vi "swabian_apply_channel_settings.vi"(8 "error in (no error)":errorcluster, 9 "Trigger edge":bool[](array[boolean])=[FALSE, FALSE, FALSE, FALSE, FALSE, FALSE, FALSE, FALSE], 10 "swabian_channel_settings":T5=[{"Threshold (V)"=0.5, "Input Delay (ps)"=0, "Dead Time (ps)"=6000}, {"Threshold (V)"=0.5, "Input Delay (ps)"=0, "Dead Time (ps)"=6000}, {"Threshold (V)"=0.5, "Input Delay (ps)"=0, "Dead Time (ps)"=6000}, {"Threshold (V)"=0.5, "Input Delay (ps)"=0, "Dead Time (ps)"=6000}, {"Threshold (V)"=0.5, "Input Delay (ps)"=0, "Dead Time (ps)"=6000}, {"Threshold (V)"=0.5, "Input Delay (ps)"=0, "Dead Time (ps)"=6000}, {"Threshold (V)"=0.5, "Input Delay (ps)"=0, "Dead Time (ps)"=6000}, {"Threshold (V)"=0.5, "Input Delay (ps)"=0, "Dead Time (ps)"=6000}] {"Dead Time (ps)" min=0 step=6000; "Input Delay (ps)" min=0 step=1; "Threshold (V)" min=0.0 max=2.5 step=0.1}, 11 "swabian_local_data":T1={"events"={"update_status"=refnum, "update_chart"=refnum, "update_xy"=refnum, "send_channel_data"=refnum}, "stop_q"=refnum, "tagger_reference"=refnum, "connect_button"=refnum, "counter_reference"=refnum, "tagger_stream_reference"=refnum, "log_reference"=refnum, "current_log_offset"=0, "tt20_buffer_q"=refnum, "stream_to_file_button"=refnum, "num_records"=0, "connected?"=FALSE, "plots"=refnum, "histogram_bin_edges"=[], "histogrammer"=refnum, "plot_lifetimes"=refnum, "xy_graph"=refnum, "Reference\nChannel"=enum."ch0", "trigger_channels"=[], "filter_channels"=[], "active_channels"=[], "acq_mode"=0, "Reference\nChannel"=enum."ch0", "acq_time"=0, "leftovers"={"leftover_stamps"=[], "leftover_channels"=[], "any?"=FALSE}, "sync_period_ps"=0, "raw_stream_path"=path "", "Leftovers"={"missing_sync_data"=[], "missing_events"=0}, "first_batch"=0, "first_sync_stamp"=0}) -> (0 "error IO":errorcluster, 3 "swabian_local_data 2":T1={"events"={"update_status"=refnum, "update_chart"=refnum, "update_xy"=refnum, "send_channel_data"=refnum}, "stop_q"=refnum, "tagger_reference"=refnum, "connect_button"=refnum, "counter_reference"=refnum, "tagger_stream_reference"=refnum, "log_reference"=refnum, "current_log_offset"=0, "tt20_buffer_q"=refnum, "stream_to_file_button"=refnum, "num_records"=0, "connected?"=FALSE, "plots"=refnum, "histogram_bin_edges"=[], "histogrammer"=refnum, "plot_lifetimes"=refnum, "xy_graph"=refnum, "Reference\nChannel"=enum."ch0", "trigger_channels"=[], "filter_channels"=[], "active_channels"=[], "acq_mode"=0, "Reference\nChannel"=enum."ch0", "acq_time"=0, "leftovers"={"leftover_stamps"=[], "leftover_channels"=[], "any?"=FALSE}, "sync_period_ps"=0, "raw_stream_path"=path "", "Leftovers"={"missing_sync_data"=[], "missing_events"=0}, "first_batch"=0, "first_sync_stamp"=0})   [LabVIEW 2018]
uses:
  swabian_channel_settings.ctl
  channel_settings.ctl
  swabian_local_data_tdef.ctl
  swabian_events_tdef.ctl
  update_chart_tdef.ctl
  channel_data_tdef.ctl
  C:/Users/SWIR TCSPC/Desktop/Swabian/lib/TTCSharp32.dll
  lib/TTCSharp32.dll
  swabian_buffer_tdef.ctl
  reference_checkbox_tdef.ctl
  leftovers_struct.ctl
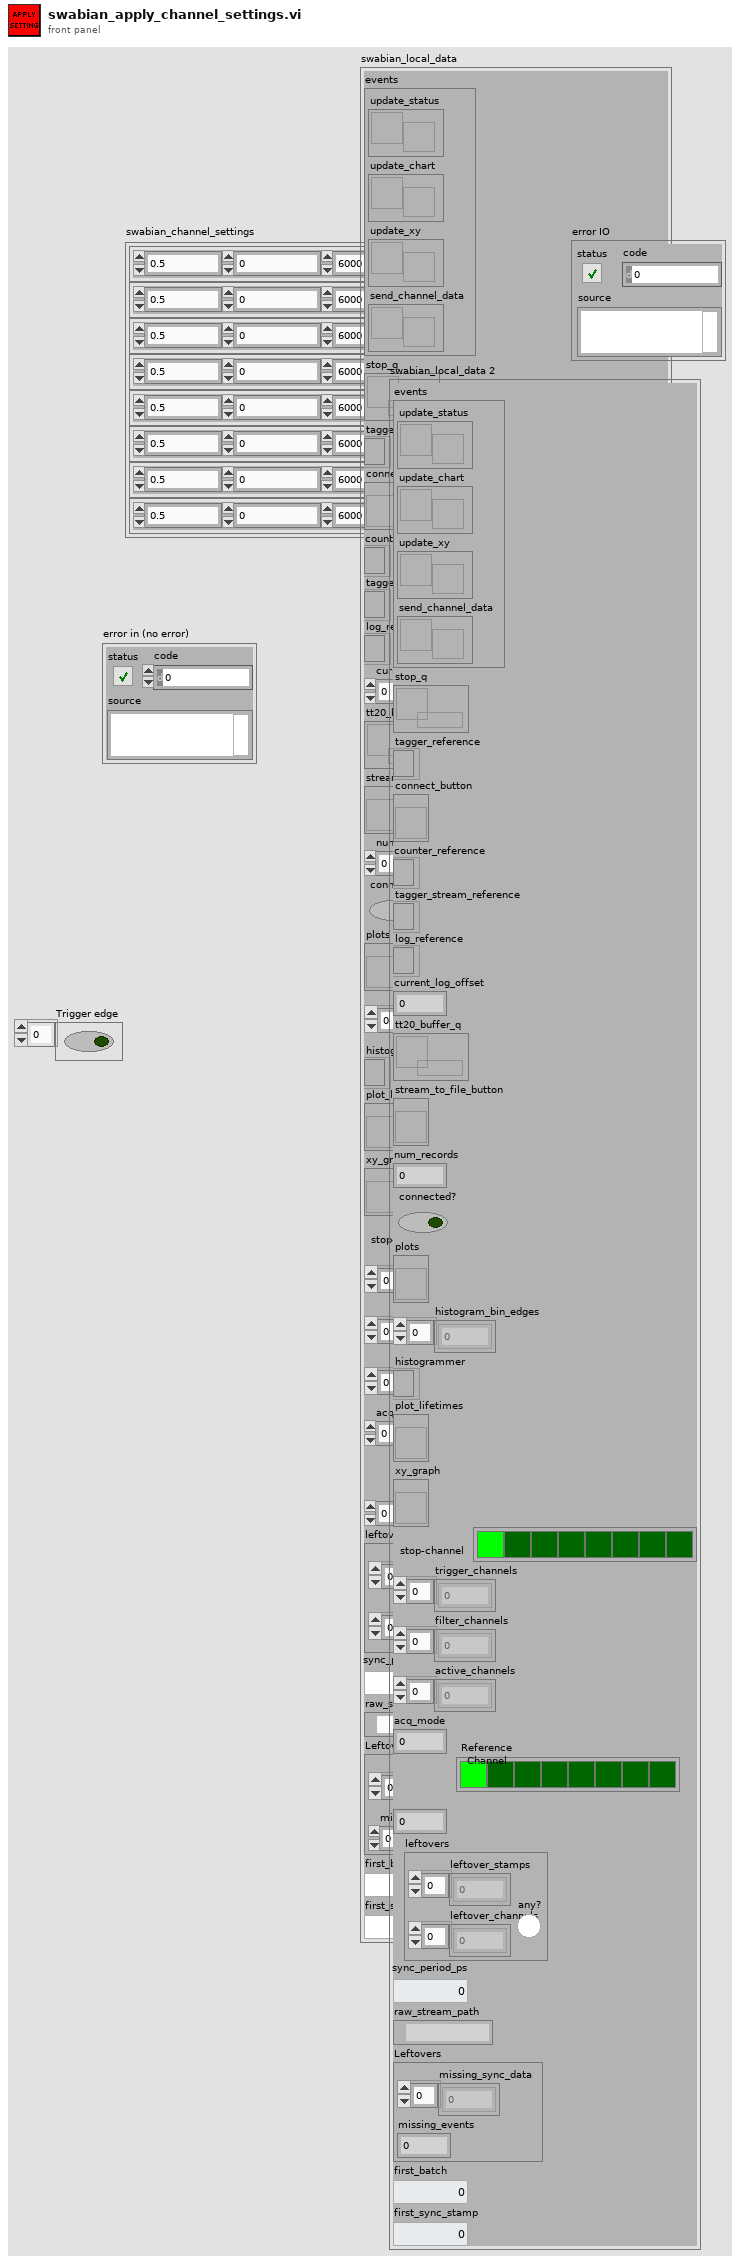
[diagram p1: front panel]
types:
  T1 = typedef "swabian_local_data_tdef.ctl" = cluster{"events":T2, "stop_q":refnum<queue>, "tagger_reference":refnum<k24>, "connect_button":refnum<vi>, "counter_reference":refnum<k24>, "tagger_stream_reference":refnum<k24>, "log_reference":refnum<file>, "current_log_offset":i64, "tt20_buffer_q":refnum<queue>, "stream_to_file_button":refnum<vi>, "num_records":u64, "connected?":bool, "plots":refnum<vi>, "histogram_bin_edges":i64[], "histogrammer":refnum<k24>, "plot_lifetimes":refnum<vi>, "xy_graph":refnum<vi>, "Reference\nChannel":T3, "trigger_channels":i32[], "filter_channels":i32[], "active_channels":i32[], "acq_mode":i32, "Reference\nChannel":T3, "acq_time":i64, "leftovers":T4, "sync_period_ps":i64, "raw_stream_path":path, "Leftovers":cluster{"missing_sync_data":u64[], "missing_events":i32}, "first_batch":i32, "first_sync_stamp":u64}
  T2 = typedef "swabian_events_tdef.ctl" = cluster{"update_status":refnum<user-event>, "update_chart":refnum<user-event>, "update_xy":refnum<user-event>, "send_channel_data":refnum<user-event>}
  T3 = typedef "reference_checkbox_tdef.ctl" = enum32{"No Selection", "ch0", "ch1", "ch2", "ch3", "ch4", "ch5", "ch6", "ch7"}
  T4 = typedef "leftovers_struct.ctl" = cluster{"leftover_stamps":i64[], "leftover_channels":i32[], "any?":bool}
  T5 = typedef "swabian_channel_settings.ctl" = T6[]
  T6 = typedef "channel_settings.ctl" = cluster{"Threshold (V)":dbl, "Input Delay (ps)":i64, "Dead Time (ps)":i64}
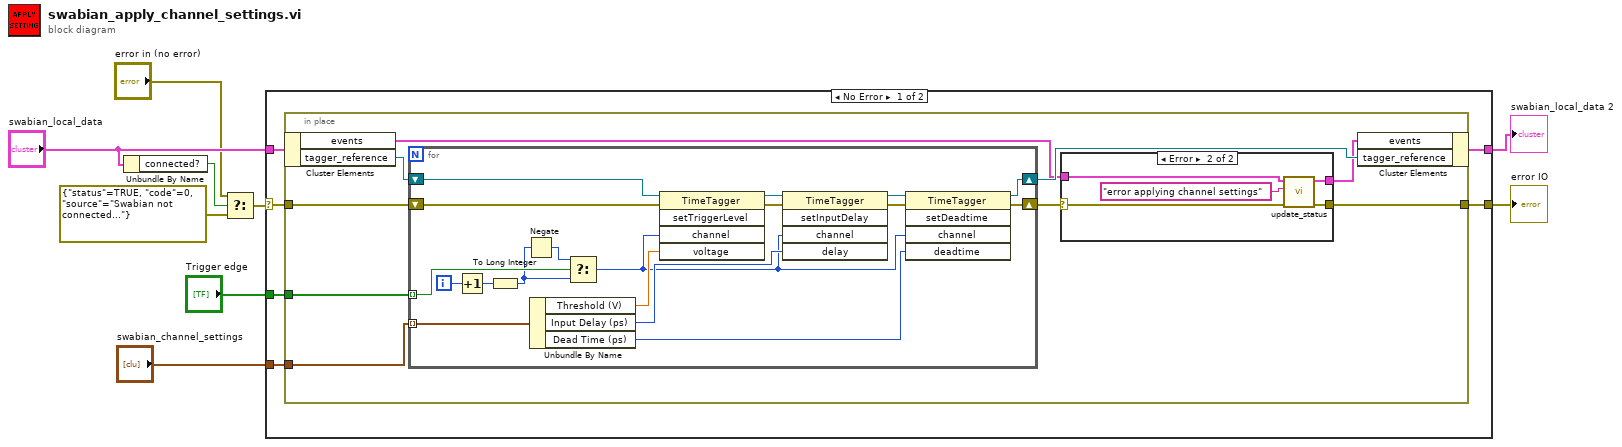
[diagram p0: block diagram]
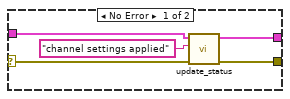
[diagram p2: hidden frame]
diagram:
  n1 = Unbundle By Name("swabian_local_data") -> ("connected?"=w5:bool)
  n2 = Select(t="error in (no error)", s=w5, f=errorcluster {"status"=TRUE, "code"=0, "source"="Swabian not connected..."}) -> (s? t:f=w3:errorcluster)
  n3 = case shown="No Error" w3 {
    selector: w3 -> [w15 w54]
    tunnel: [w14 w54] -> w9
    tunnel: "swabian_channel_settings" -> [w13 _]
    tunnel: "swabian_local_data" -> [w12 w53]
    tunnel: [w11 w53] -> w7
    tunnel: "Trigger edge" -> [w10 _]
    frame No Error {
      n4 = in-place {
        in-place-border: w15 -> [w24]
        in-place-border: [w17] -> w14
        in-place-border: w13 -> [w23]
        in-place-border: w10 -> [w16]
        n5 = in-place-cluster #1(w12) -> ("events"=w19:T2, "tagger_reference"=w22:refnum<k24>)
        n6 = for {
          shift-right: [w47] -> w20
          shift-left: w24 -> [w48]
          tunnel: w23 -> [w46] mode=indexing
          shift-right: [w41] -> w21
          shift-left: w22 -> [w42]
          tunnel: w16 -> [w38] mode=indexing
          i -> [w40]
          n7 = Increment(x=w40) -> (x+1=w39:i32)
          n8 = To Long Integer(number=w39) -> (32bit integer=w35:i32)
          n9 = Negate(x=w35) -> (-x=w36:i32)
          n10 = Unbundle By Name(w46) -> ("Threshold (V)"=w45:dbl, "Input Delay (ps)"=w44:i64, "Dead Time (ps)"=w43:i64)
          n11 = Select(t=w36, s=w38, f=w35) -> (s? t:f=w37:i32)
          n12 = invoke class="TimeTagger" method="setTriggerLevel"(reference=w42, error in=w48, "channel"=w37, "voltage"=w45) -> (reference out=w52:refnum<k24>, error out=w51:errorcluster)  [unwired: 1 in, 3 out]
          n13 = invoke class="TimeTagger" method="setInputDelay"(reference=w52, error in=w51, "channel"=w37, "delay"=w44) -> (reference out=w50:refnum<k24>, error out=w49:errorcluster)  [unwired: 1 in, 3 out]
          n14 = invoke class="TimeTagger" method="setDeadtime"(reference=w50, error in=w49, "channel"=w37, "deadtime"=w43) -> (reference out=w41:refnum<k24>, error out=w47:errorcluster)  [unwired: 1 in, 3 out]
        }
        n15 = case shown="Error" w20 {
          selector: w20 -> [w29 w32]
          tunnel: w19 -> [w28 w34]
          tunnel: [w27 w33] -> w18
          tunnel: [w26 w31] -> w17
          frame No Error {
            n16 = call "update_status.vi"("error in (no error)"=w29, "status"="channel settings applied", "events"=w28) -> ("error out"=w26:errorcluster, "events_out"=w27:T2)  [unwired: 7 in]
          }
          frame Error {
            n17 = call "update_status.vi"("error in (no error)"=w32, "status"="error applying channel settings", "events"=w34) -> ("error out"=w31:errorcluster, "events_out"=w33:T2)  [unwired: 7 in]
          }
        }
        n18 = in-place-cluster #1("events"=w18, "tagger_reference"=w21) -> (w11:T1)
      }
    }
    frame Error {
    }
  }
  "error IO" <- w9
  "swabian_local_data 2" <- w7
